vi "Configure Websockets Connection.vi"(6 "timeout (5000 ms)":i32=5000, 8 "error in (no error)":errorcluster, 9 "path":string, 10 "remote port (80)":u16=80, 11 "address (localhost)":string="localhost") -> (0 "error out":errorcluster, 3 "WSConnection":refnum<class "WebsocketsConnection.lvclass">)   [LabVIEW 2013, in "MQTT_Websockets.lvlib" / "WebsocketsConnection.lvclass"]
uses:
  WebsocketsConnection.lvclass
  WebsocketsConnection.lvclass/WebsocketsConnection.ctl
  MQTT_Connection/Connection/Connection.lvclass/Connection.ctl
  MQTT_Connection/Connection/Connection.lvclass
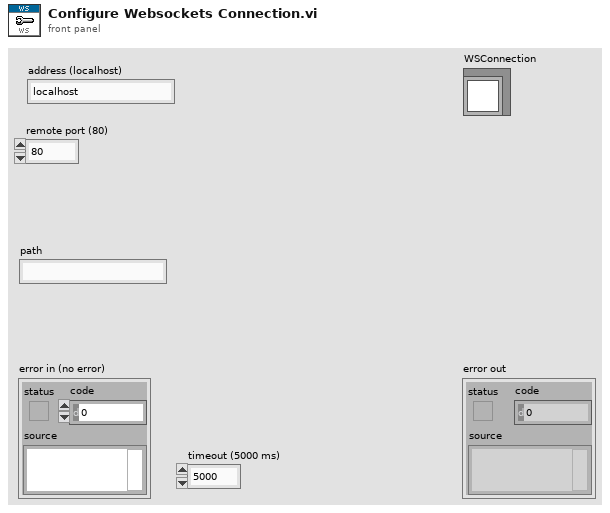
[diagram p1: front panel]
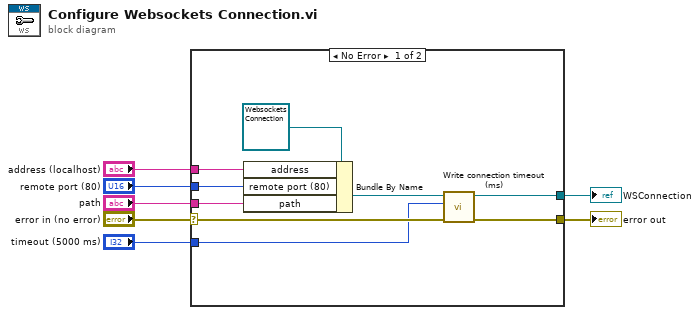
[diagram p0: block diagram]
diagram:
  n1 = case shown="No Error" "error in (no error)" {
    selector: "error in (no error)" -> [w12 w17]
    tunnel: [w9 w17] -> w6
    tunnel: [w10 _] -> w2
    tunnel: "address (localhost)" -> [w15 _]
    tunnel: "remote port (80)" -> [w14 _]
    tunnel: "timeout (5000 ms)" -> [w11 _]
    tunnel: "path" -> [w8 _]
    frame No Error {
      n2 = Bundle By Name(cluster=refnum<class "WebsocketsConnection.lvclass"> refnum ("TCPConnection in"), "address"=w15, "remote port (80)"=w14, "path"=w8) -> (w13:refnum<class "WebsocketsConnection.lvclass">)
      n3 = call "Write connection timeout (ms).vi"("error in (no error)"=w12, "connection timeout (ms)"=w11, "Connection in"=w13) -> ("error out"=w9:errorcluster, "Connection out"=w10:refnum<class "WebsocketsConnection.lvclass">)  [unwired: 7 in]
    }
    frame Error {
    }
  }
  "error out" <- w6
  "WSConnection" <- w2
